vi "HB CH2 radius.vi"(8 "error in":errorcluster) -> (0 "error out":errorcluster, 2 "CH2 found?":bool)   [LabVIEW 2021, in "Component Tray.lvclass"]
uses:
  Component Tray.lvclass
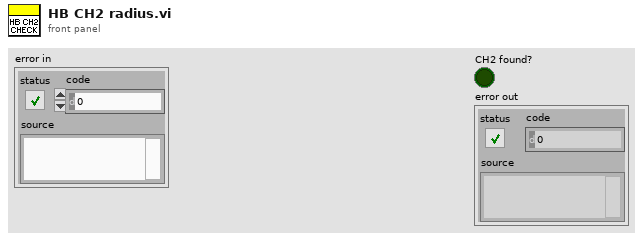
[diagram p1: front panel]
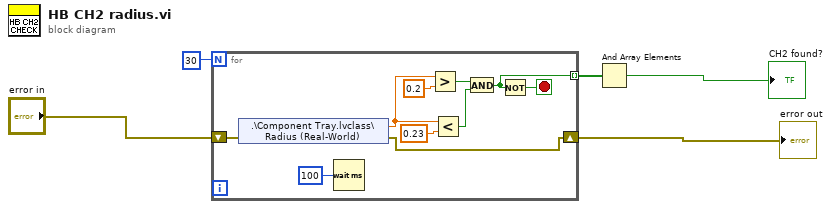
[diagram p0: block diagram]
diagram:
  n1 = for {
    N: 30 -> [_]
    tunnel: [w7] -> w3 mode=indexing
    shift-right: [w10] -> w5
    shift-left: "error in" -> [w9]
    stop <- w8 stop-if-true
    n2 = shared-variable ".\\Component Tray.lvclass\\Radius (Real-World)"(error in=w9) -> (w15:dbl, error out=w10:errorcluster)
    n3 = Wait (ms)(milliseconds to wait=u32 100) -> ()  [unwired: 1 out]
    n4 = Greater?(x=w15, y=0.2) -> (0:w11:bool)
    n5 = Less?(x=w15, y=0.23) -> (x < y?=w12:bool)
    n6 = And(x=w11, y=w12) -> (x .and. y?=w7:bool)
    n7 = Not(x=w7) -> (.not. x?=w8:bool)
  }
  "error out" <- w5
  n8 = And Array Elements(Boolean array=w3) -> (logical AND=→"CH2 found?":bool)
